vi "ROI group-Search group names.vi"(9 "Group names to search for":string[](array[string]), 11 "Group names to search through":string[](array[string])) -> (3 "Indexes (-1 = not found)":i32[](array[numeric]))   [LabVIEW 2017]
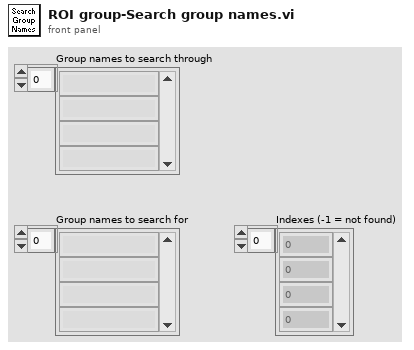
[diagram p1: front panel]
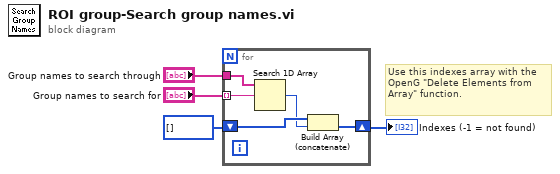
[diagram p0: block diagram]
diagram:
  # "Use this indexes array with the OpenG \"Delete Elements from Array\" function."
  n1 = for {
    tunnel: "Group names to search through" -> [w9]
    tunnel: "Group names to search for" -> [w8] mode=indexing
    shift-right: [w7] -> w1
    shift-left: i32[] [] -> [w6]
    n2 = Search 1D Array(1D array=w9, element=w8) -> (index of element=w5:i32)  [unwired: 1 in]
    n3 = Build Array (concatenate)(w6, w5) -> (w7:i32[])
  }
  "Indexes (-1 = not found)" <- w1
